vi "GetGreatestCube.vi"(8 "error in (no error)":errorcluster, 11 "S4GUI in":refnum<class "S4GUI.lvclass">) -> (0 "error out":errorcluster, 3 "S4GUI out":refnum<class "S4GUI.lvclass">, 4 "greatest (ms)":dbl)   [LabVIEW 2018, in "S4GUI.lvclass"]
uses:
  S4GUI.lvclass
  S4GUI.lvclass/S4GUI.ctl
  Acquisition/Acquisition.lvclass
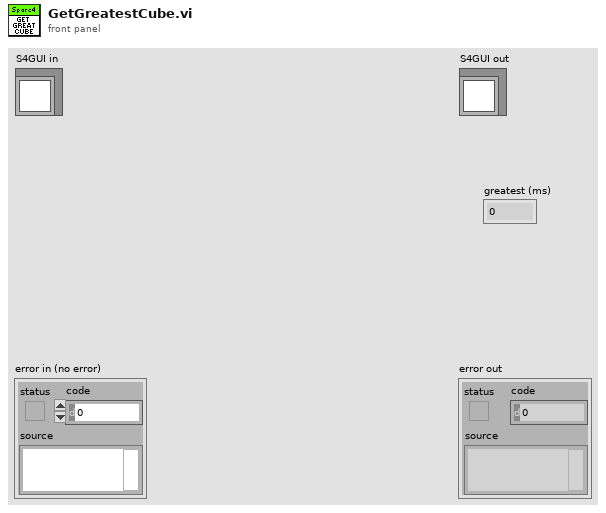
[diagram p1: front panel]
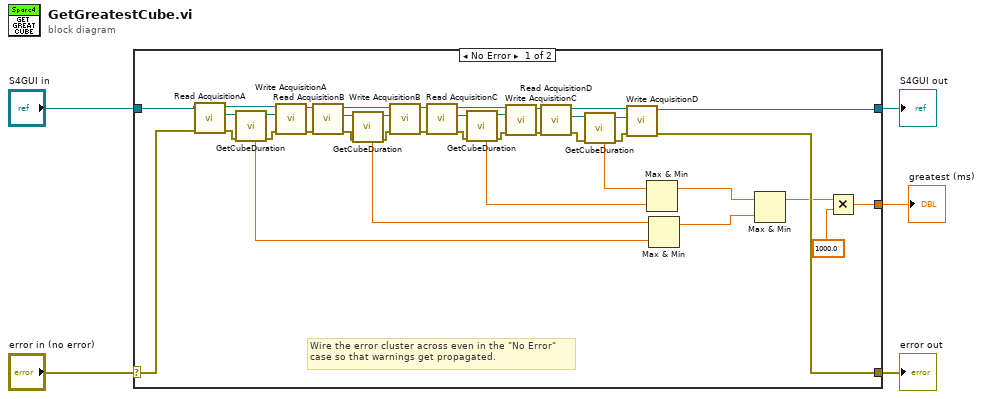
[diagram p0: block diagram]
diagram:
  n1 = case shown="No Error" "error in (no error)" {
    selector: "error in (no error)" -> [w10 w46]
    tunnel: [w9 w46] -> w4
    tunnel: [w17 w45] -> w2
    tunnel: "S4GUI in" -> [w18 w45]
    tunnel: [w6 _] -> w1
    frame No Error {
      # "Wire the error cluster across even in the \"No Error\"\ncase so that warnings get propagated."
      n2 = call-dynamic "Read AcquisitionA.vi"("error in (no error)"=w10, "S4ACS_GUI in"=w18) -> ("error out"=w37:errorcluster, "Acquisition.lvclass"=w31:refnum<class "Acquisition.lvclass">, "S4ACS_GUI out"=w44:refnum<class "S4GUI.lvclass">)  [unwired: 7 in]
      n3 = call-dynamic "GetCubeDuration.vi"("error in (no error)"=w37, "Acquisition in"=w31) -> ("error out"=w36:errorcluster, "Acquisition out"=w30:refnum<class "Acquisition.lvclass">, "CubeDuration"=w11:dbl)  [unwired: 7 in]
      n4 = call-dynamic "Write AcquisitionA.vi"("error in (no error)"=w36, "Acquisition.lvclass"=w30, "S4ACS_GUI in"=w44) -> ("error out"=w35:errorcluster, "S4ACS_GUI out"=w43:refnum<class "S4GUI.lvclass">)  [unwired: 7 in]
      n5 = call "Read AcquisitionB.vi"("error in (no error)"=w35, "S4ACS_GUI in"=w43) -> ("error out"=w34:errorcluster, "Acquisition.lvclass"=w29:refnum<class "Acquisition.lvclass">, "S4ACS_GUI out"=w42:refnum<class "S4GUI.lvclass">)  [unwired: 7 in]
      n6 = call-dynamic "GetCubeDuration.vi"("error in (no error)"=w34, "Acquisition in"=w29) -> ("error out"=w33:errorcluster, "Acquisition out"=w28:refnum<class "Acquisition.lvclass">, "CubeDuration"=w12:dbl)  [unwired: 7 in]
      n7 = call "Write AcquisitionB.vi"("error in (no error)"=w33, "Acquisition.lvclass"=w28, "S4ACS_GUI in"=w42) -> ("error out"=w32:errorcluster, "S4ACS_GUI out"=w41:refnum<class "S4GUI.lvclass">)  [unwired: 7 in]
      n8 = call-dynamic "Read AcquisitionC.vi"("error in (no error)"=w32, "S4ACS_GUI in"=w41) -> ("error out"=w23:errorcluster, "Acquisition.lvclass"=w27:refnum<class "Acquisition.lvclass">, "S4ACS_GUI out"=w40:refnum<class "S4GUI.lvclass">)  [unwired: 7 in]
      n9 = call-dynamic "GetCubeDuration.vi"("error in (no error)"=w23, "Acquisition in"=w27) -> ("error out"=w22:errorcluster, "Acquisition out"=w26:refnum<class "Acquisition.lvclass">, "CubeDuration"=w13:dbl)  [unwired: 7 in]
      n10 = call-dynamic "Write AcquisitionC.vi"("error in (no error)"=w22, "Acquisition.lvclass"=w26, "S4ACS_GUI in"=w40) -> ("error out"=w21:errorcluster, "S4ACS_GUI out"=w39:refnum<class "S4GUI.lvclass">)  [unwired: 7 in]
      n11 = call-dynamic "Read AcquisitionD.vi"("error in (no error)"=w21, "S4ACS_GUI in"=w39) -> ("error out"=w20:errorcluster, "Acquisition.lvclass"=w25:refnum<class "Acquisition.lvclass">, "S4ACS_GUI out"=w38:refnum<class "S4GUI.lvclass">)  [unwired: 7 in]
      n12 = call-dynamic "GetCubeDuration.vi"("error in (no error)"=w20, "Acquisition in"=w25) -> ("error out"=w19:errorcluster, "Acquisition out"=w24:refnum<class "Acquisition.lvclass">, "CubeDuration"=w14:dbl)  [unwired: 7 in]
      n13 = call-dynamic "Write AcquisitionD.vi"("error in (no error)"=w19, "Acquisition.lvclass"=w24, "S4ACS_GUI in"=w38) -> ("error out"=w9:errorcluster, "S4ACS_GUI out"=w17:refnum<class "S4GUI.lvclass">)  [unwired: 7 in]
      n14 = Max & Min(x=w14, y=w13) -> (max(x,y)=w16:dbl)  [unwired: 1 out]
      n15 = Max & Min(x=w12, y=w11) -> (max(x,y)=w15:dbl)  [unwired: 1 out]
      n16 = Max & Min(x=w16, y=w15) -> (max(x,y)=w8:dbl)  [unwired: 1 out]
      n17 = Multiply(x=w8, y=1000.0) -> (x*y=w6:dbl)
    }
    frame Error {
    }
  }
  "error out" <- w4
  "S4GUI out" <- w2
  "greatest (ms)" <- w1
